vi "PWM Write.vi"(7 "PWM line":T1=1700 items=["Port0/DIO4 (Left Motor)"=1004, "Port0/DIO5 (Right Motor)"=1005, "Port0/DIO7 (Servo)"=1007, "Port7/DIO0"=1700, "Port7/DIO1"=1701, "Port7/DIO2"=1702, "Port7/DIO3"=1703], 8 "error in (no error)":errorcluster, 9 "pulse width (us)":u32=1500, 10 "period (us)":u32=20000, 11 "direct IO in":refnum<class "NI_Robotics_Starter Kit Direct IO.lvclass">) -> (0 "error out":errorcluster, 3 "direct IO out":refnum<class "NI_Robotics_Starter Kit Direct IO.lvclass">)   [LabVIEW 2017, in "NI_Robotics_Starter Kit Direct IO.lvclass"]
uses:
  <vilib>/robotics/Starter Kit/Direct IO/NI_Robotics_Starter Kit Direct IO.lvclass
  <vilib>/robotics/Starter Kit/Direct IO/PWM Lines.ctl
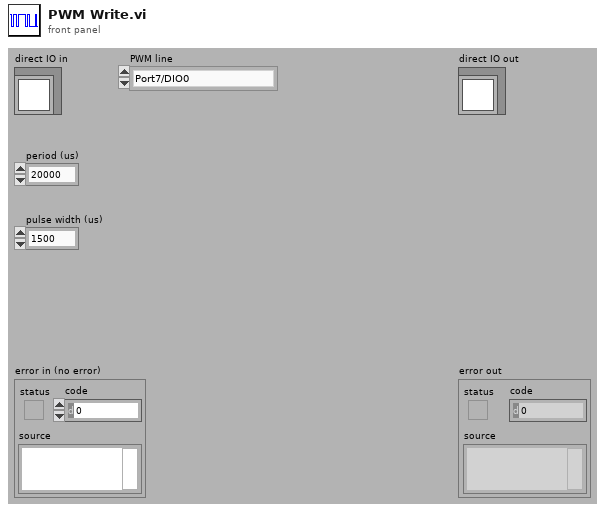
[diagram p1: front panel]
types:
  T1 = typedef "NI_Robotics_Starter Kit Direct IO.lvclass/PWM Lines.ctl" = u16
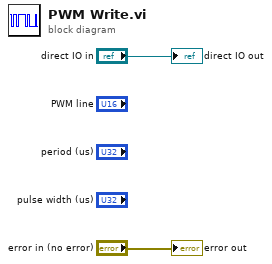
[diagram p0: block diagram]
diagram:
  "error out" <- "error in (no error)"
  "direct IO out" <- "direct IO in"
